vi "Check Loop Error.vi"(6 "Quitter en cas d'erreur ? (F)":bool, 9 "Ignorer les erreurs":i32[](array[numeric]), 10 "erreur à traiter":T1, 11 "File d'attente de messages":refnum<queue>) -> (2 "Erreur ?":bool, 3 "File d'attente de message dup.":refnum<queue>)   [LabVIEW 2018]
doc: "Vérifier l'erreur à traiter pour voir si sa valeur de code correspond à une des valeurs du tableau 'Erreurs à ignorer'. Si c'est le cas, ne rien faire. Sinon, envoyer un message \"Error\" contenant les données de l'erreur à la boucle de gestion de messages pour un traitement supplémentaire. Mais si l'entrée \"Quitter en cas d'erreur\" est VRAI, envoyer un message \"Exit\" à la boucle de gestion de messages."
uses:
  Message Queue/Message Cluster.ctl
  Message Queue/Enqueue Message (Single).vi
  Message Queue/Message Queue.lvlib
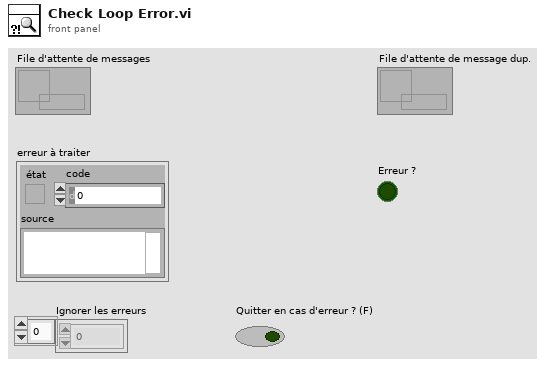
[diagram p1: front panel]
types:
  T1 = cluster{"état":bool, "code":i32, "source":string}
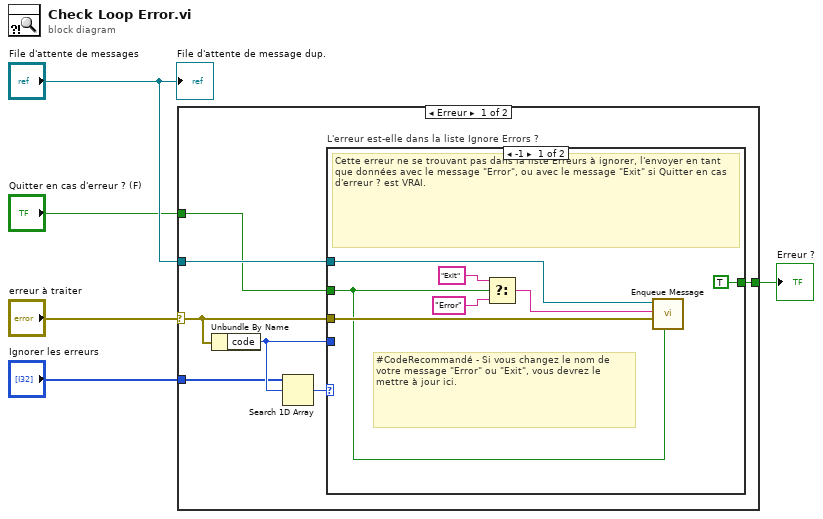
[diagram p0: block diagram]
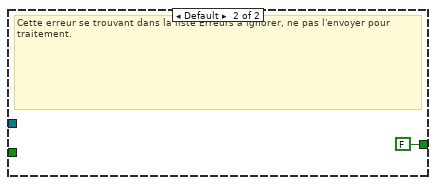
[diagram p2: hidden frame]
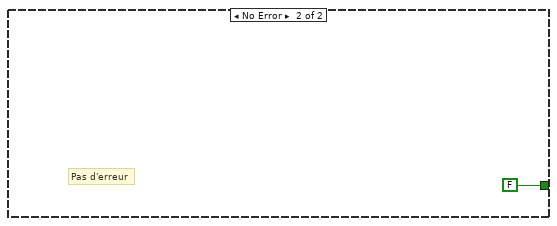
[diagram p3: hidden frame]
diagram:
  n1 = case shown="Erreur" "erreur à traiter" {
    selector: "erreur à traiter" -> [w9 _]
    tunnel: "File d'attente de messages" -> [w12 _]
    tunnel: "Ignorer les erreurs" -> [w8 _]
    tunnel: [w7 FALSE] -> w2
    tunnel: "Quitter en cas d'erreur ? (F)" -> [w6 _]
    frame Error {
      n2 = Unbundle By Name(w9) -> ("code"=w10:i32)
      n3 = Search 1D Array(1D array=w8, element=w10) -> (index of element=w11:i32)  [unwired: 1 in]
      n4 = case "L'erreur est-elle dans la liste Ignore Errors ?" shown="-1" w11 {
        tunnel: w9 -> [w17 _]
        tunnel: w12 -> [w19 _]
        tunnel: w10 -> [_ _]
        tunnel: [TRUE FALSE] -> w7
        tunnel: w6 -> [w16 _]
        frame -1 {
          # "#CodeRecommandé - Si vous changez le nom de votre message \"Error\" ou \"Exit\", vous devrez le mettre à jour ici."
          # "Cette erreur ne se trouvant pas dans la liste Erreurs à ignorer, l'envoyer en tant que données avec le message \"Error\", ou avec le message \"Exit\" si Quitter en cas d'erreur ? est VRAI."
          n5 = Select(t="Exit" ("Message"), s=w16, f="Error" ("Message")) -> (s? t:f=w15:string)
          n6 = call-poly "Enqueue Message.vi"("Message prioritaire ? (F)"=w16, "Données de message"=w17, "Message"=w15, "File d'attente de messages"=w19) -> ()  [unwired: 6 in, 2 out]
        }
        frame Default {
          # "Cette erreur se trouvant dans la liste Erreurs à ignorer, ne pas l'envoyer pour traitement."
        }
      }
    }
    frame No Error {
      # "Pas d'erreur"
    }
  }
  "Erreur ?" <- w2
  "File d'attente de message dup." <- "File d'attente de messages"
